vi "SlowQDKS2020+-Post-Uninstall.vi"(10 "Variant":variant) -> (0 "error out":errorcluster)   [LabVIEW 2020]
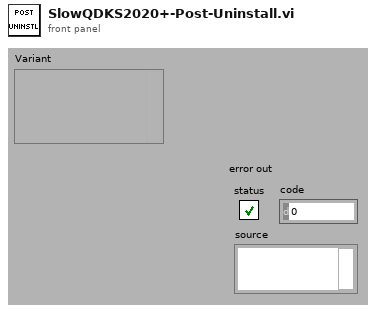
[diagram p1: front panel]
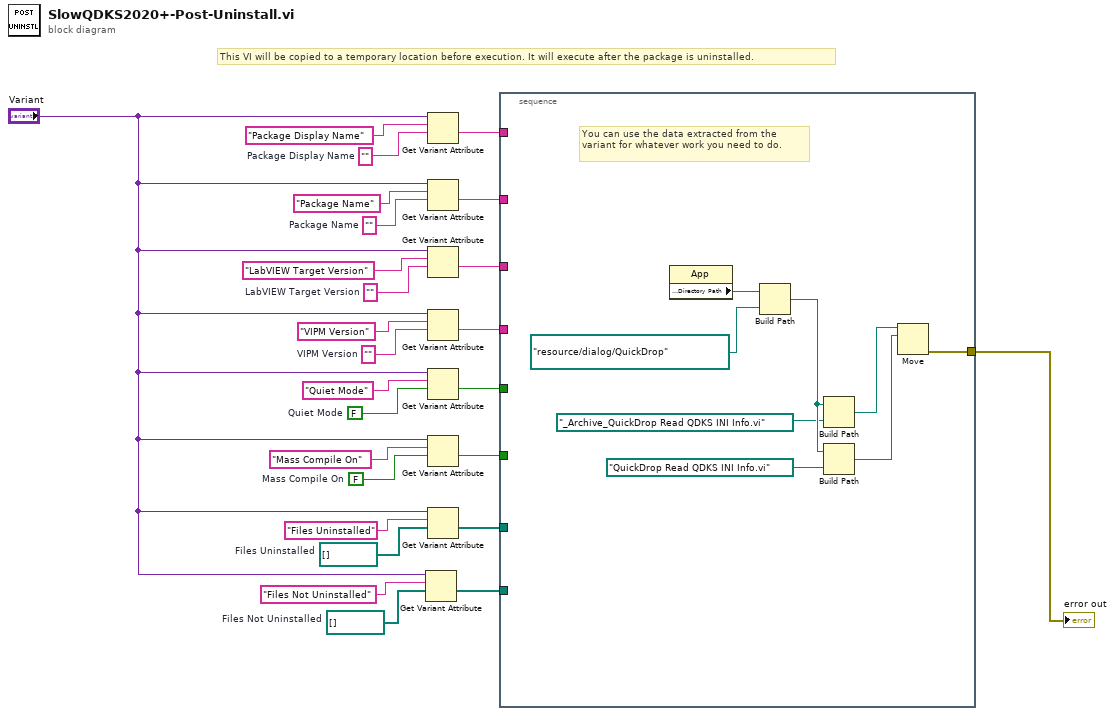
[diagram p0: block diagram]
diagram:
  w2 = path[] []  # Files Not Uninstalled
  w3 = path[] []  # Files Uninstalled
  w9 = FALSE  # Mass Compile On
  w10 = ""  # Package Display Name
  w17 = FALSE  # Quiet Mode
  w20 = ""  # VIPM Version
  w22 = ""  # LabVIEW Target Version
  w24 = ""  # Package Name
  # "This VI will be copied to a temporary location before execution. It will execute after the package is uninstalled."
  n1 = Get Variant Attribute(Variant="Variant", name="Files Not Uninstalled", default value (empty Variant)=w2) -> (value=w7:path[])  [unwired: 1 in, 3 out]
  n2 = Get Variant Attribute(Variant="Variant", name="Package Display Name", default value (empty Variant)=w10) -> (value=w16:string)  [unwired: 1 in, 3 out]
  n3 = Get Variant Attribute(Variant="Variant", name="Package Name", default value (empty Variant)=w24) -> (value=w15:string)  [unwired: 1 in, 3 out]
  n4 = Get Variant Attribute(Variant="Variant", name="LabVIEW Target Version", default value (empty Variant)=w22) -> (value=w14:string)  [unwired: 1 in, 3 out]
  n5 = Get Variant Attribute(Variant="Variant", name="VIPM Version", default value (empty Variant)=w20) -> (value=w13:string)  [unwired: 1 in, 3 out]
  n6 = Get Variant Attribute(Variant="Variant", name="Quiet Mode", default value (empty Variant)=w17) -> (value=w12:bool)  [unwired: 1 in, 3 out]
  n7 = Get Variant Attribute(Variant="Variant", name="Mass Compile On", default value (empty Variant)=w9) -> (value=w11:bool)  [unwired: 1 in, 3 out]
  n8 = Get Variant Attribute(Variant="Variant", name="Files Uninstalled", default value (empty Variant)=w3) -> (value=w6:path[])  [unwired: 1 in, 3 out]
  n9 = stacked-sequence {
    tunnel: w16 -> [_]
    tunnel: w15 -> [_]
    tunnel: w14 -> [_]
    tunnel: w13 -> [_]
    tunnel: w12 -> [_]
    tunnel: w11 -> [_]
    tunnel: w6 -> [_]
    tunnel: w7 -> [_]
    tunnel: [w29] -> w1
    frame #0 {
      # "You can use the data extracted from the variant for whatever work you need to do."
      n10 = property class="App"() -> ("Application:Directory Path"=w34:path)  [unwired: 2 in, 2 out]
      n11 = Build Path(base path=w34, name or relative path=path "resource/dialog/QuickDrop") -> (appended path=w32:path)
      n12 = Build Path(base path=w32, name or relative path=path "_Archive_QuickDrop Read QDKS INI Info.vi") -> (appended path=w31:path)
      n13 = Build Path(base path=w32, name or relative path=path "QuickDrop Read QDKS INI Info.vi") -> (appended path=w30:path)
      n14 = Move(source path=w31, 10:w30) -> (error out=w29:errorcluster)  [unwired: 3 in, 2 out]
    }
  }
  "error out" <- w1
